vi "SaveWriteSetupFile.vi"(8 "Error In":errorcluster, 10 "Setup":T1={"DUT"={"Count"=1, "Wirings"=[], "Names"=[]}, "Log"={"Start"={"Trigger Type"=enum."Immediate", "Timer (sec)"=0.0, "Digital IO Line"=0, "Digital IO Edge"=enum."Rising"}, "Rollover"={"Trigger Type"=enum."None", "Timer (sec)"=0.0, "File Size (MB)"=0, "Digital IO Line"=0, "Digital IO Edge"=enum."Rising"}, "Stop"={"Trigger Type"=enum."None", "Timer (sec)"=0.0, "File Size (MB)"=0, "Digital IO Line"=0, "Digital IO Edge"=enum."Rising"}}, "Trigger"={"Input"={"Type"=enum."None", "Timeout (ms)"=0, "Delay (ms)"=0, "Digital IO Line (1-14)"=0, "Digital IO Mode"=enum."Falling"}, "Output"={"Type"=enum."None", "Delay (ms)"=0, "Digital IO Line (1-14)"=0, "Digital IO Mode"=enum."Falling", "Digital IO Pulse Width (sec)"=0.0}}, "Sources"=[], "Measures"=[]} {"Measures"."Count" min=1 step=1; "Trigger"."Output"."Digital IO Line (1-14)" min=1 max=14 step=1}, 11 "Save File":path) -> (0 "Error Out":errorcluster)   [LabVIEW 2012]
uses:
  Setup.ctl
  DUTConfiguration.ctl
  driver/Public/Controls/SMUSense.ctl
  LogConfiguration.ctl
  LogStartConfiguration.ctl
  LogStartTriggerType.ctl
  LogDigitalIOTriggerEdge.ctl
  LogRolloverConfiguration.ctl
  LogRolloverTriggerType.ctl
  LogStopConfiguration.ctl
  LogStopTriggerType.ctl
  TriggerConfiguration.ctl
  TriggerInputConfiguration.ctl
  TriggerInputType.ctl
  driver/Public/Controls/TriggerMode.ctl
  TriggerOutputConfiguration.ctl
  TriggerOutputType.ctl
  SourceConfiguration.ctl
  SourceFunction.ctl
  MeasureConfiguration.ctl
  <vilib>/xml/Close Reference(Node).vi
  <vilib>/xml/NI_XML.lvlib
  <resource>/objmgr/DOMUserDefRef.rc
  libs/LV-Utilities/LV-Utilities.lvlib
  driver/Keithley-2602.lvlib
panel:
  out "XML":string
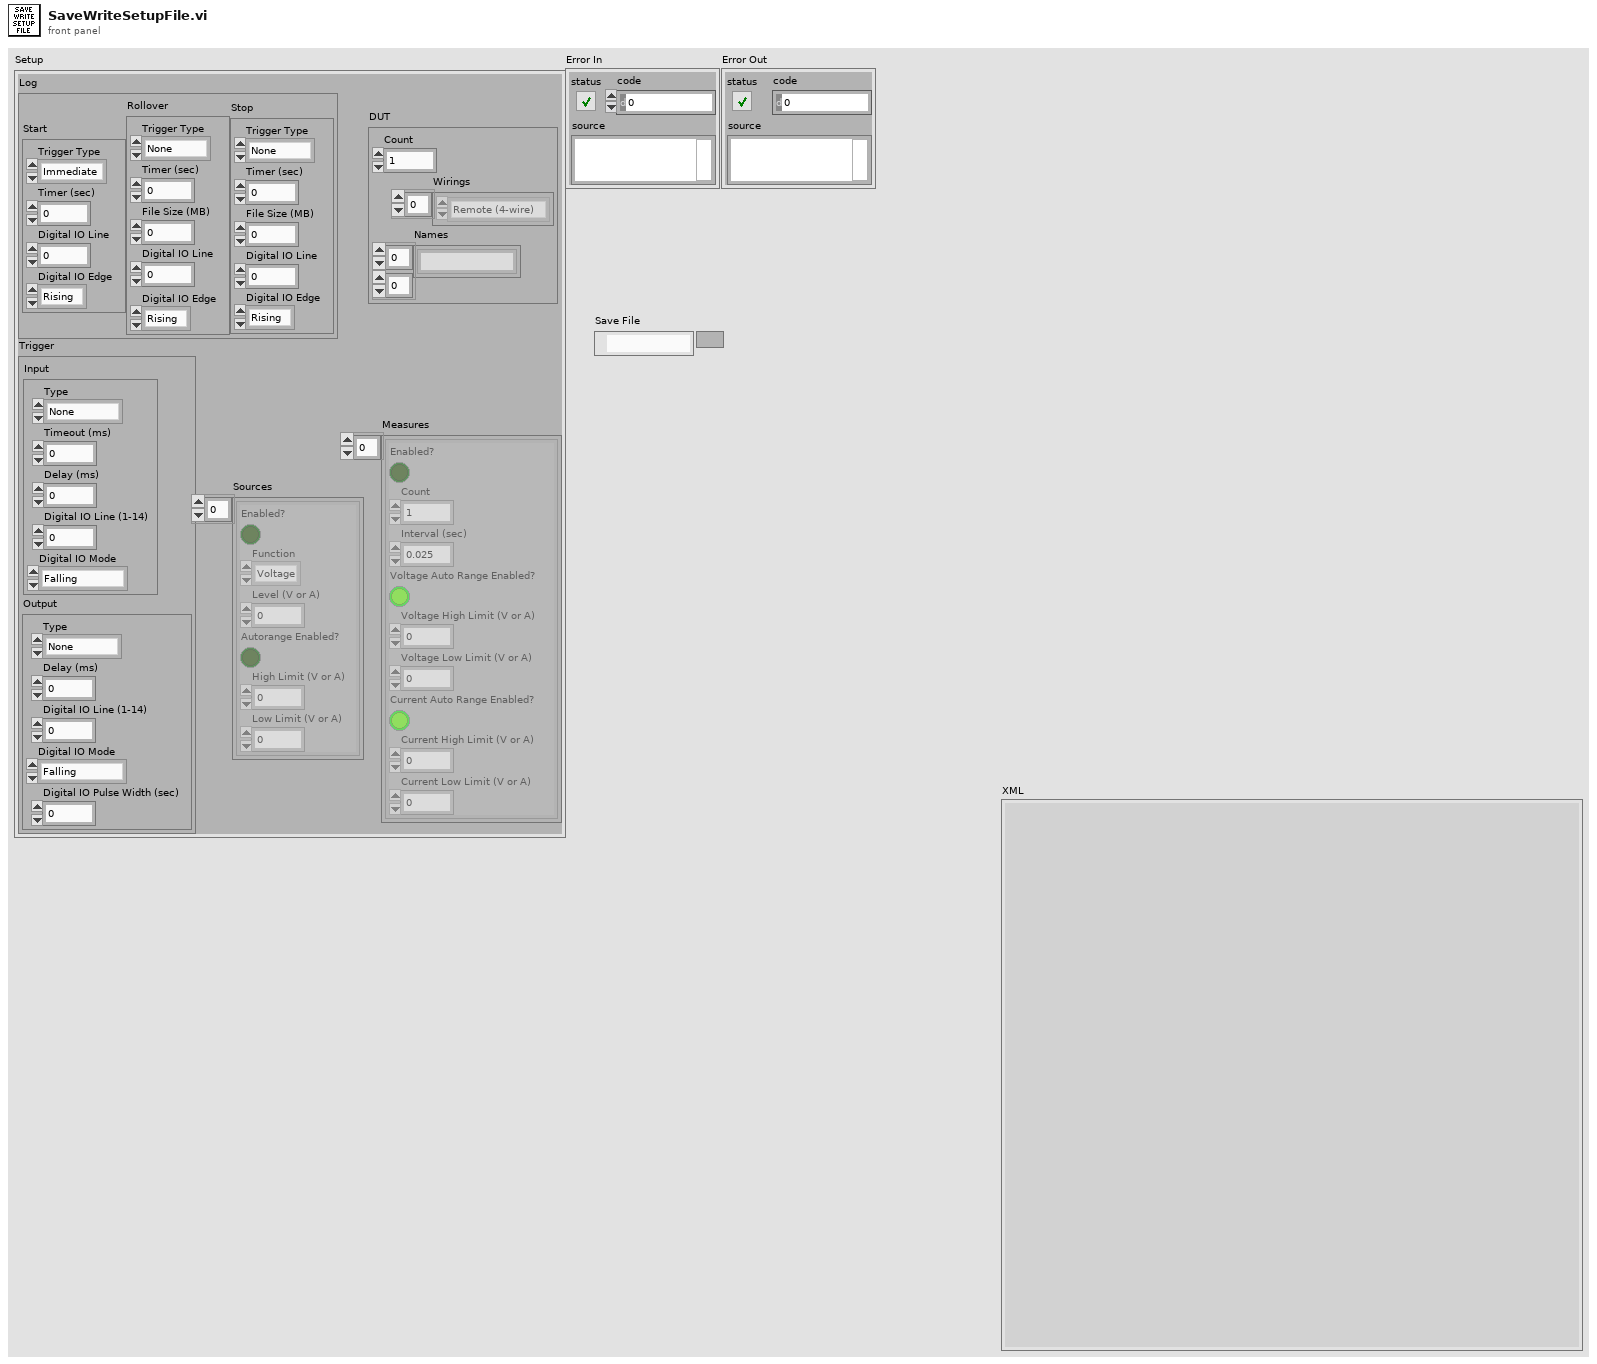
[diagram p1: front panel]
types:
  T1 = typedef "Setup.ctl" = cluster{"DUT":T2, "Log":T4, "Trigger":T12, "Sources":T18[], "Measures":T20[]}
  T2 = typedef "DUTConfiguration.ctl" = cluster{"Count":u32, "Wirings":T3[], "Names":string[][]}
  T3 = typedef "Keithley-2602.lvlib/SMUSense.ctl" = enum16{"Local (2-wire)", "Remote (4-wire)", "Calibration"}
  T4 = typedef "LogConfiguration.ctl" = cluster{"Start":T5, "Rollover":T8, "Stop":T10}
  T5 = typedef "LogStartConfiguration.ctl" = cluster{"Trigger Type":T6, "Timer (sec)":dbl, "Digital IO Line":u8, "Digital IO Edge":T7}
  T6 = typedef "LogStartTriggerType.ctl" = enum16{"Immediate", "User", "Timer", "Digital IO"}
  T7 = typedef "LogDigitalIOTriggerEdge.ctl" = enum16{"Rising", "Falling"}
  T8 = typedef "LogRolloverConfiguration.ctl" = cluster{"Trigger Type":T9, "Timer (sec)":dbl, "File Size (MB)":u32, "Digital IO Line":u8, "Digital IO Edge":T7}
  T9 = typedef "LogRolloverTriggerType.ctl" = enum16{"None", "Timer", "File Size", "Digital IO"}
  T10 = typedef "LogStopConfiguration.ctl" = cluster{"Trigger Type":T11, "Timer (sec)":dbl, "File Size (MB)":u32, "Digital IO Line":u8, "Digital IO Edge":T7}
  T11 = typedef "LogStopTriggerType.ctl" = enum16{"None", "User", "Timer", "File Size", "Digital IO"}
  T12 = typedef "TriggerConfiguration.ctl" = cluster{"Input":T13, "Output":T16}
  T13 = typedef "TriggerInputConfiguration.ctl" = cluster{"Type":T14, "Timeout (ms)":u32, "Delay (ms)":u32, "Digital IO Line (1-14)":u8, "Digital IO Mode":T15}
  T14 = typedef "TriggerInputType.ctl" = enum16{"None", "Digital IO", "Bus"}
  T15 = typedef "Keithley-2602.lvlib/TriggerMode.ctl" = enum16{"Falling", "Rising", "Either", "Synchronous"}
  T16 = typedef "TriggerOutputConfiguration.ctl" = cluster{"Type":T17, "Delay (ms)":u32, "Digital IO Line (1-14)":u8, "Digital IO Mode":T15, "Digital IO Pulse Width (sec)":dbl}
  T17 = typedef "TriggerOutputType.ctl" = enum16{"None", "Digital IO", "Bus"}
  T18 = typedef "SourceConfiguration.ctl" = cluster{"Enabled?":bool, "Function":T19, "Level (V or A)":dbl, "Autorange Enabled?":bool, "High Limit (V or A)":dbl, "Low Limit (V or A)":dbl}
  T19 = typedef "SourceFunction.ctl" = enum16{"Voltage", "Current"}
  T20 = typedef "MeasureConfiguration.ctl" = cluster{"Enabled?":bool, "Count":u8, "Interval (sec)":dbl, "Voltage Auto Range Enabled?":bool, "Voltage High Limit (V or A)":dbl, "Voltage Low Limit (V or A)":dbl, "Current Auto Range Enabled?":bool, "Current High Limit (V or A)":dbl, "Current Low Limit (V or A)":dbl}
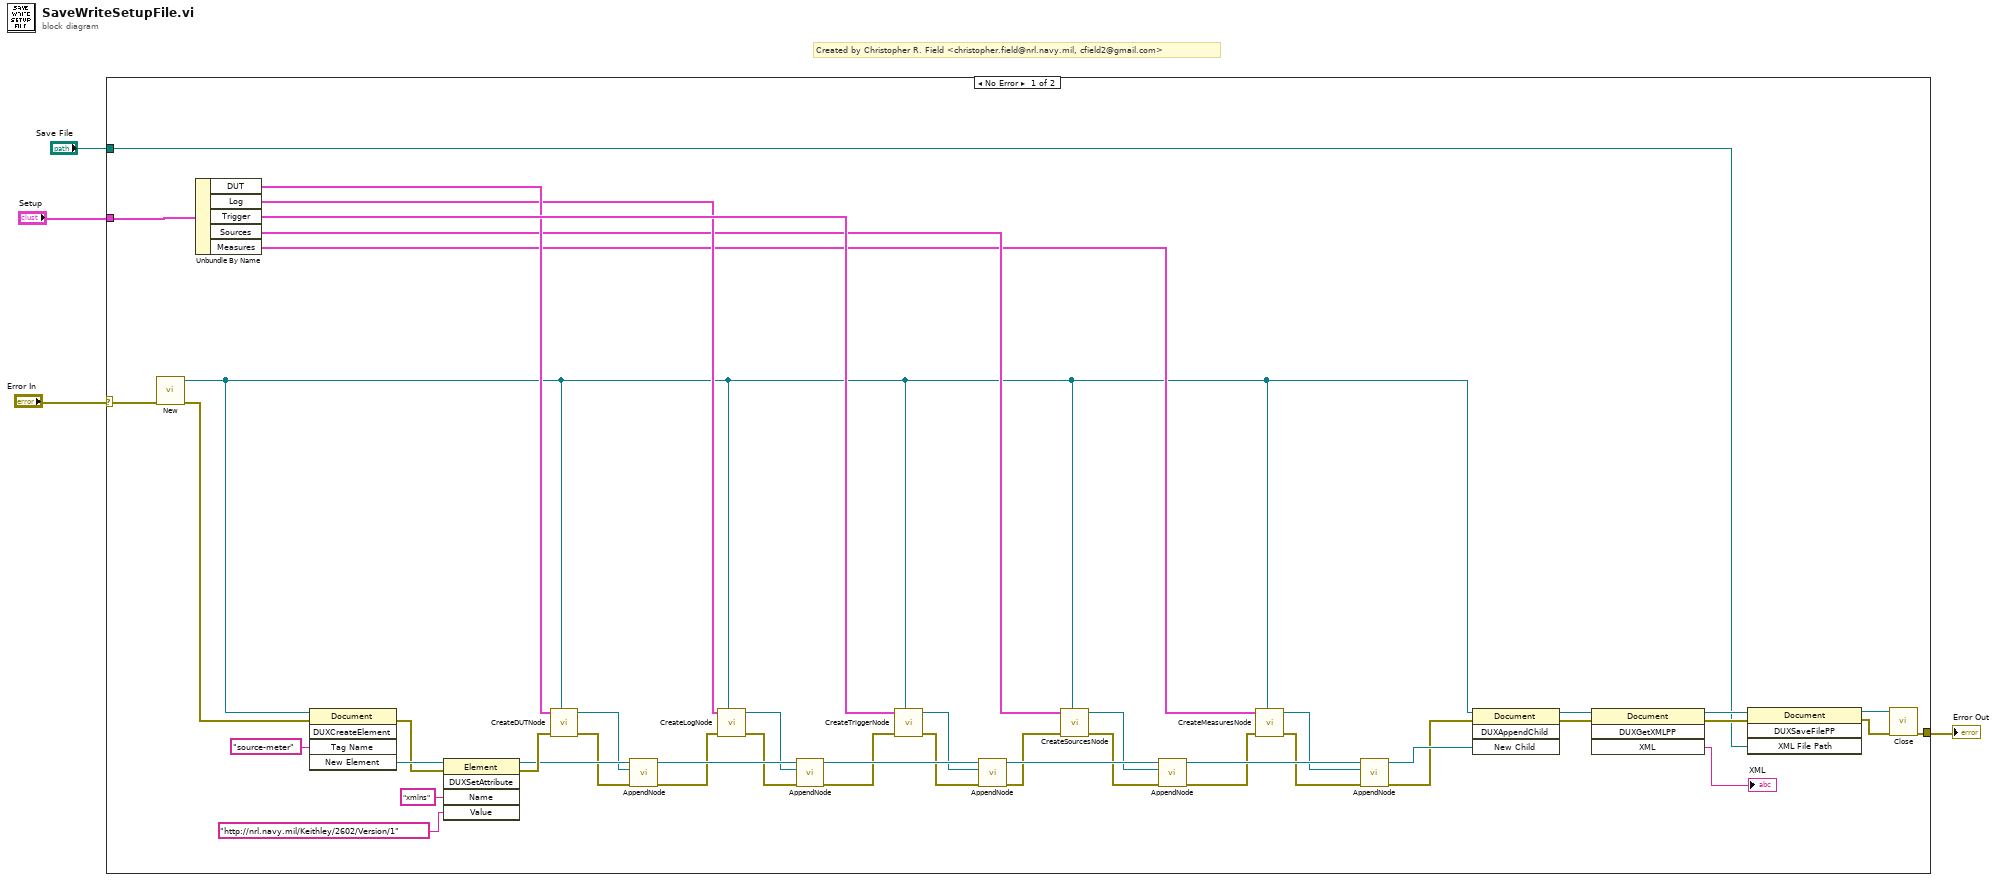
[diagram p0: block diagram]
diagram:
  # "Created by Christopher R. Field <christopher.field@nrl.navy.mil, cfield2@gmail.com>"
  n1 = case shown="No Error" "Error In" {
    selector: "Error In" -> [w49 w50]
    tunnel: "Setup" -> [w22 _]
    tunnel: "Save File" -> [w42 _]
    tunnel: [w43 w50] -> w1
    frame No Error {
      n2 = call <vilib>:"New.vi"("error in (no error)"=w49) -> ("error out"=w36:errorcluster, "DOM document out"=w6:refnum<k20>)  [unwired: 7 in]
      n3 = Unbundle By Name(w22) -> ("DUT"=w19:T2, "Log"=w15:T4, "Trigger"=w21:T12, "Sources"=w10:T18[], "Measures"=w7:T20[])
      n4 = invoke class="Document" method="DUXCreateElement"(reference=w6, error in=w36, "Tag Name"="source-meter") -> (error out=w39:errorcluster, "New Element"=w40:refnum<k20>)  [unwired: 2 in, 3 out]
      n5 = invoke class="Element" method="DUXSetAttribute"(reference=w40, error in=w39, "Name"="xmlns", "Value"="http://nrl.navy.mil/Keithley/2602/Version/1") -> (reference out=w32:refnum<k20>, error out=w35:errorcluster)  [unwired: 1 in, 3 out]
      n6 = call "CreateDUTNode.vi"("DOM Document"=w6, "Error In"=w35, "DUT Configuration"=w19) -> ("Error Out"=w17:errorcluster, "DUT Node"=w18:refnum<k20>)  [unwired: 7 in]
      n7 = call "AppendNode.vi"("Error In"=w17, "Child Node"=w18, "Parent Node In"=w32) -> ("Error Out"=w16:errorcluster, "Parent Node Out"=w31:refnum<k20>)  [unwired: 7 in]
      n8 = call "CreateLogNode.vi"("DOM Document"=w6, "Error In"=w16, "Log Configuration"=w15) -> ("Error Out"=w13:errorcluster, "Log Node"=w14:refnum<k20>)  [unwired: 7 in]
      n9 = call "AppendNode.vi"("Error In"=w13, "Child Node"=w14, "Parent Node In"=w31) -> ("Error Out"=w20:errorcluster, "Parent Node Out"=w30:refnum<k20>)  [unwired: 7 in]
      n10 = call "CreateTriggerNode.vi"("DOM Document"=w6, "Error In"=w20, "Trigger Configuration"=w21) -> ("Error Out"=w23:errorcluster, "Trigger Node"=w24:refnum<k20>)  [unwired: 7 in]
      n11 = call "AppendNode.vi"("Error In"=w23, "Child Node"=w24, "Parent Node In"=w30) -> ("Error Out"=w12:errorcluster, "Parent Node Out"=w29:refnum<k20>)  [unwired: 7 in]
      n12 = call "CreateSourcesNode.vi"("DOM Document"=w6, "Error In"=w12, "Sources"=w10) -> ("Error Out"=w11:errorcluster, "Sources Node"=w9:refnum<k20>)  [unwired: 7 in]
      n13 = call "AppendNode.vi"("Error In"=w11, "Child Node"=w9, "Parent Node In"=w29) -> ("Error Out"=w8:errorcluster, "Parent Node Out"=w28:refnum<k20>)  [unwired: 7 in]
      n14 = call "CreateMeasuresNode.vi"("DOM Document"=w6, "Error In"=w8, "Measures"=w7) -> ("Error Out"=w25:errorcluster, "Measures Node"=w5:refnum<k20>)  [unwired: 7 in]
      n15 = call "AppendNode.vi"("Error In"=w25, "Child Node"=w5, "Parent Node In"=w28) -> ("Error Out"=w26:errorcluster, "Parent Node Out"=w27:refnum<k20>)  [unwired: 7 in]
      n16 = invoke class="Document" method="DUXAppendChild"(reference=w6, error in=w26, "New Child"=w27) -> (reference out=w34:refnum<k20>, error out=w33:errorcluster)  [unwired: 1 in, 2 out]
      n17 = invoke class="Document" method="DUXGetXMLPP"(reference=w34, error in=w33) -> (reference out=w48:refnum<k20>, error out=w47:errorcluster, "XML"=→"XML":string)  [unwired: 2 in, 1 out]
      n18 = invoke class="Document" method="DUXSaveFilePP"(reference=w48, error in=w47, "XML File Path"=w42) -> (reference out=w46:refnum<k20>, error out=w45:errorcluster)  [unwired: 1 in, 2 out]
      n19 = call-poly <vilib>:"Close.vi"("error in (no error)"=w45, "node"=w46) -> ("error out"=w43:errorcluster)  [unwired: 7 in]
    }
    frame Error {
    }
  }
  "Error Out" <- w1
